vi "Get_State_INI_.vi"(0 "Application_Directory":path, 11 "Error_In":errorcluster) -> (4 "Data":string, 15 "Error_Out":errorcluster)   [LabVIEW 2023]
doc: "This VI get the state data from the ini file."
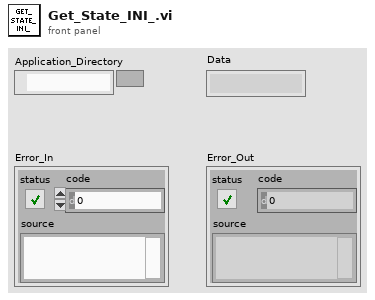
[diagram p1: front panel]
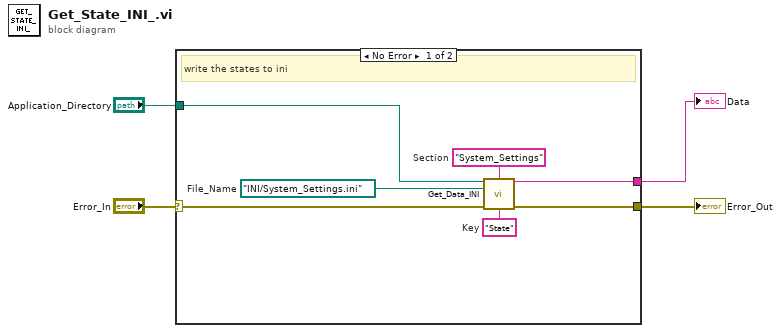
[diagram p0: block diagram]
diagram:
  n1 = case shown="No Error" "Error_In" {
    selector: "Error_In" -> [w8 w12]
    tunnel: "Application_Directory" -> [w11 _]
    tunnel: [w9 w12] -> w3
    tunnel: [w5 _] -> w1
    frame No Error {
      w7 = "State"  # Key
      w6 = "System_Settings"  # Section
      w10 = path "INI/System_Settings.ini"  # File_Name
      # "write the states to ini"
      n2 = call "Get_Data_INI.vi"("Application_Directory"=w11, "Section"=w6, "File_Name"=w10, "Error_In"=w8, "Key"=w7) -> ("Data"=w5:string, "Error_Out"=w9:errorcluster)  [unwired: 9 in]
    }
    frame Error {
    }
  }
  "Error_Out" <- w3
  "Data" <- w1
